vi "Read Status Active_NonActive.vi"(8 "error in (no error)":errorcluster, 11 "GeneralFunctionality in":refnum<class "GeneralFunctionality.lvclass">) -> (0 "error out":errorcluster, 2 "Status Active/NonActive":bool, 3 "GeneralFunctionality out":refnum<class "GeneralFunctionality.lvclass">)   [LabVIEW 2020, in "GeneralFunctionality.lvclass"]
uses:
  GeneralFunctionality.lvclass
  GeneralFunctionality.lvclass/GeneralFunctionality.ctl
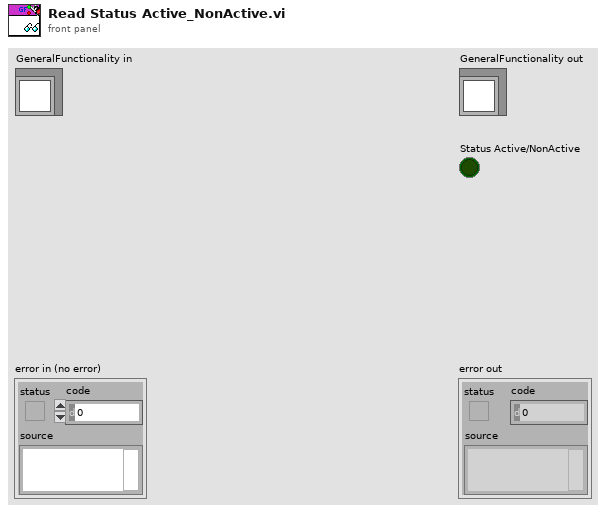
[diagram p1: front panel]
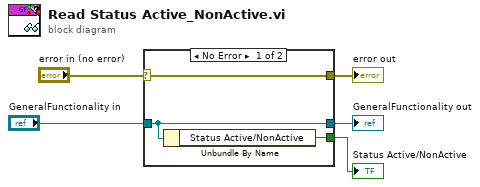
[diagram p0: block diagram]
diagram:
  n1 = case shown="No Error" "error in (no error)" {
    selector: "error in (no error)" -> [w8 w9]
    tunnel: [w8 w9] -> w4
    tunnel: [w7 w10] -> w2
    tunnel: "GeneralFunctionality in" -> [w7 w10]
    tunnel: [w6 _] -> w1
    frame No Error {
      n2 = Unbundle By Name(w7) -> ("Status Active/NonActive"=w6:bool)
    }
    frame Error {
    }
  }
  "error out" <- w4
  "GeneralFunctionality out" <- w2
  "Status Active/NonActive" <- w1
